vi "Status Pump Status.vi"(5 "Retry Attempts (0)":i32 min=0, 8 "error in (no error)":errorcluster, 11 "VISA resource name":refnum<visa-resource-name>) -> (0 "error out":errorcluster, 2 "Status Cluster":T1, 3 "VISA resource name out":refnum<visa-resource-name>)   [LabVIEW 2020, in "ChromTech Series III Pump.lvlib"]
doc: "Returns the current pump information."
uses:
  <instrlib>/RxnRover/ChromtechSeriesIIIDriver/ChromTech Series III Pump.lvlib
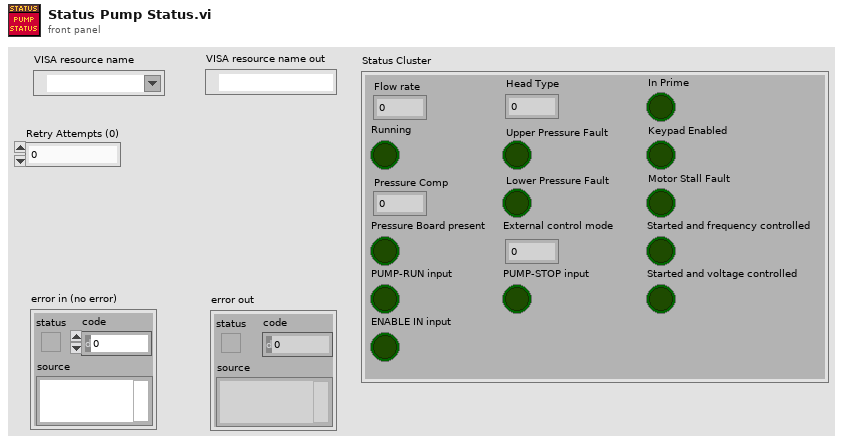
[diagram p1: front panel]
types:
  T1 = cluster{"Flow rate":dbl, "Running":bool, "Pressure Comp":i32, "Head Type":i32, "Upper Pressure Fault":bool, "Lower Pressure Fault":bool, "In Prime":bool, "Keypad Enabled":bool, "Motor Stall Fault":bool, "Pressure Board present":bool, "External control mode":i32, "Started and frequency controlled":bool, "Started and voltage controlled":bool, "PUMP-RUN input":bool, "PUMP-STOP input":bool, "ENABLE IN input":bool}
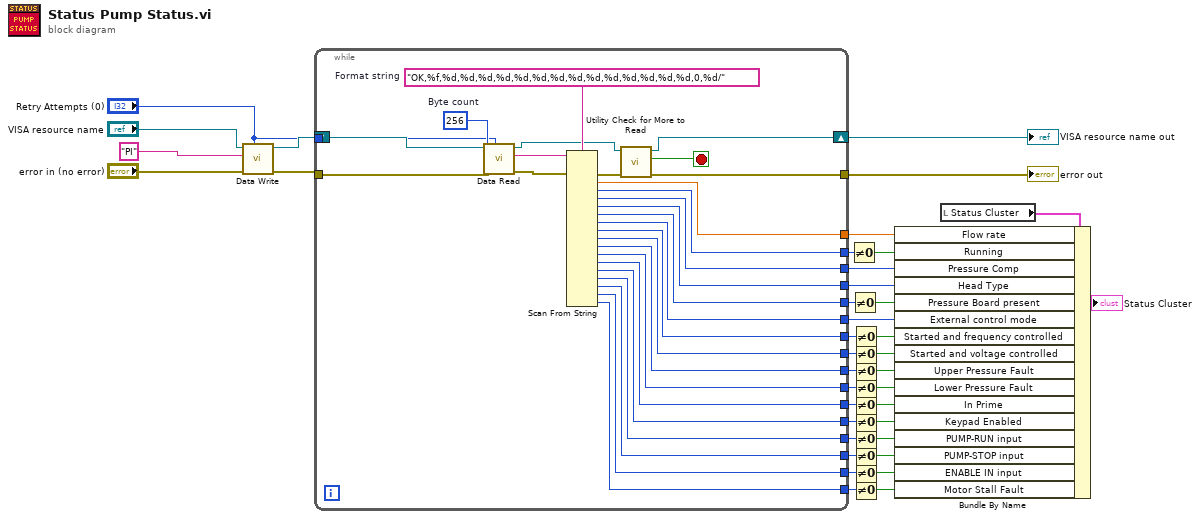
[diagram p0: block diagram]
diagram:
  n1 = call <instrlib>:"Data Write.vi"("Retry Attempts (0)"="Retry Attempts (0)", "error in (no error)"="error in (no error)", "Command"="PI" ("command"), "VISA Refnum in"="VISA resource name") -> ("error out"=w3:errorcluster, "VISA Refnum out"=w2:refnum<visa-resource-name>)  [unwired: 6 in]
  n2 = while {
    tunnel: [w65] -> w34
    tunnel: [w64] -> w32
    tunnel: [w63] -> w31
    tunnel: [w62] -> w30
    tunnel: [w58] -> w26
    tunnel: [w57] -> w25
    tunnel: [w56] -> w14
    tunnel: [w55] -> w13
    tunnel: [w54] -> w12
    tunnel: [w53] -> w11
    tunnel: [w52] -> w10
    tunnel: [w51] -> w9
    tunnel: [w50] -> w8
    tunnel: [w49] -> w7
    tunnel: [w48] -> w6
    tunnel: [w47] -> w5
    tunnel: "Retry Attempts (0)" -> [w43]
    shift-right: [w40] -> w29
    shift-left: w2 -> [w44]
    tunnel: w3 -> [w46]
    tunnel: [w42] -> w28
    stop <- w39 stop-if-true
    w45 = u32 256  # Byte count
    w66 = "OK,%f,%d,%d,%d,%d,%d,%d,%d,%d,%d,%d,%d,%d,%d,%d,0,%d/"  # Format string
    n3 = call <instrlib>:"Data Read.vi"("Retry Attempts (0)"=w43, "error in (no error)"=w46, "Bytes to read"=w45, "VISA Refnum in"=w44) -> ("error out"=w61:errorcluster, "read buffer"=w59:string, "VISA Refnum out"=w41:refnum<visa-resource-name>)  [unwired: 5 in]
    n4 = Scan From String(format string=w66, input string=w59, error in=w61) -> (error out=w60:errorcluster, output 1=w65:dbl, output 2=w64:i32, output 3=w63:i32, output 4=w62:i32, output 5=w58:i32, output 6=w57:i32, output 7=w56:i32, output 8=w54:i32, output 9=w55:i32, output 10=w53:i32, output 11=w52:i32, output 12=w51:i32, output 13=w50:i32, output 14=w49:i32, output 15=w48:i32, output 16=w47:i32)  [unwired: 17 in, 2 out]
    n5 = call <instrlib>:"Utility Check for More to Read.vi"("error in (no error)"=w60, "VISA Refnum in"=w41) -> ("error out (unchanged)"=w42:errorcluster, "More to read?"=w39:bool, "VISA Refnum out"=w40:refnum<visa-resource-name>)  [unwired: 7 in]
  }
  "VISA resource name out" <- w29
  "error out" <- w28
  n6 = Not Equal To 0?(x=w32) -> (x != 0?=w33:bool)
  n7 = Not Equal To 0?(x=w26) -> (x != 0?=w27:bool)
  n8 = Not Equal To 0?(x=w14) -> (x != 0?=w24:bool)
  n9 = Not Equal To 0?(x=w12) -> (x != 0?=w23:bool)
  n10 = Not Equal To 0?(x=w13) -> (x != 0?=w22:bool)
  n11 = Not Equal To 0?(x=w11) -> (x != 0?=w21:bool)
  n12 = Not Equal To 0?(x=w10) -> (x != 0?=w20:bool)
  n13 = Not Equal To 0?(x=w9) -> (x != 0?=w15:bool)
  n14 = Not Equal To 0?(x=w8) -> (x != 0?=w16:bool)
  n15 = Not Equal To 0?(x=w7) -> (x != 0?=w17:bool)
  n16 = Not Equal To 0?(x=w6) -> (x != 0?=w19:bool)
  n17 = Not Equal To 0?(x=w5) -> (x != 0?=w18:bool)
  n18 = local read "Status Cluster"() -> (w36:T1)
  n19 = Bundle By Name(cluster=w36, "Flow rate"=w34, "Running"=w33, "Pressure Comp"=w31, "Head Type"=w30, "Pressure Board present"=w27, "External control mode"=w25, "Started and frequency controlled"=w24, "Started and voltage controlled"=w23, "Upper Pressure Fault"=w22, "Lower Pressure Fault"=w21, "In Prime"=w20, "Keypad Enabled"=w15, "PUMP-RUN input"=w16, "PUMP-STOP input"=w17, "ENABLE IN input"=w19, "Motor Stall Fault"=w18) -> (→"Status Cluster":T1)
